vi "Create ADOResult.vi"(8 "error in (no error)":errorcluster, 11 "Reader":refnum<k24>) -> (0 "error out":errorcluster, 3 "ADOResult out":refnum<class "ADOResult.lvclass">)   [LabVIEW 2020, in "ORM_ADONet.lvlib" / "ADOResult.lvclass"]
uses:
  ADOResult.lvclass
  System.Data
  ADOResult.lvclass/ADOResult.ctl
  Write Reader.vi
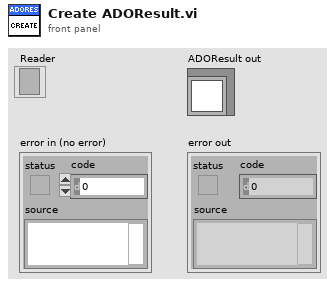
[diagram p1: front panel]
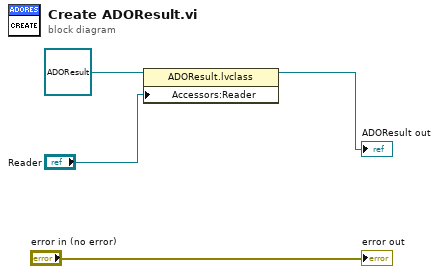
[diagram p0: block diagram]
diagram:
  n1 = property class="ADOResult.lvclass"(reference=refnum<class "ADOResult.lvclass"> refnum ("ADOResult out"), "Accessors:Reader"="Reader") -> (reference out=→"ADOResult out":refnum<class "ADOResult.lvclass">)  [unwired: 1 in, 1 out]
  "error out" <- "error in (no error)"
